vi "Are string arrays equal.vi"(8 "error in (no error)":errorcluster, 10 "1D String Array 2":string[](array[string]), 11 "1D String Array 1":string[](array[string])) -> (0 "error out":errorcluster, 3 "EQUAL?":bool)   [LabVIEW 2012]
doc: "SciScan 1.2 160622\nChecks if 2 string arrays are equal and returs a boolean (TRUE if equal; FALSE otherwise)"
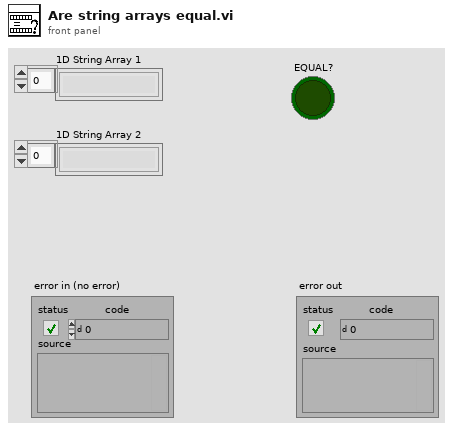
[diagram p1: front panel]
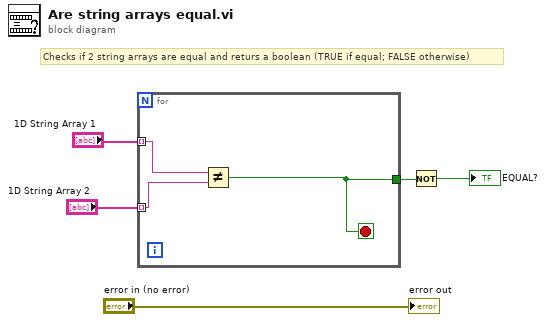
[diagram p0: block diagram]
diagram:
  # "Checks if 2 string arrays are equal and returs a boolean (TRUE if equal; FALSE otherwise)"
  n1 = for {
    tunnel: "1D String Array 2" -> [w8] mode=indexing
    tunnel: "1D String Array 1" -> [w7] mode=indexing
    tunnel: [w6] -> w5
    stop <- w6 stop-if-true
    n2 = Not Equal?(x=w7, y=w8) -> (x != y?=w6:bool)
  }
  n3 = Not(x=w5) -> (.not. x?=→"EQUAL?":bool)
  "error out" <- "error in (no error)"
